vi "Test FFT time.vi"() -> ()   [LabVIEW 2018]
uses:
  General/type defines/FFT parameters.ctl
  <vilib>/Analysis/4window.llb/windowTd.ctl
  <vilib>/Analysis/NI_AALPro.lvlib
panel:
  out "Waveform Chart":sgl[][](graph)
  in  "error in (no error)":errorcluster
  out "time for FFT":dbl
  in  "FFT parameters":T1={"window"=1, "view"={"dB On (F)"=FALSE, "unwrap phase (F)"=FALSE, "convert to degree (F)"=FALSE}, "#A-lines"=2048, "start pixel"=0, "#pixels to save"=300} {"window" items=["Rectangle"=0, "Hanning"=1, "Hamming"=2, "Blackman-Harris"=3, "Exact Blackman"=4, "Blackman"=5, "Flat Top"=6, "4 Term B-Harris "=7, "7 Term B-Harris"=8, "Low Sidelobe"=9, "Blackman Nuttall"=11, "Triangle"=30, "Bartlett-Hanning"=31, "Bohman"=32, "Parzen"=33, "Welch"=34, "Kaiser"=60, "Dolph-Chebyshev"=61, "Gaussian"=62]}
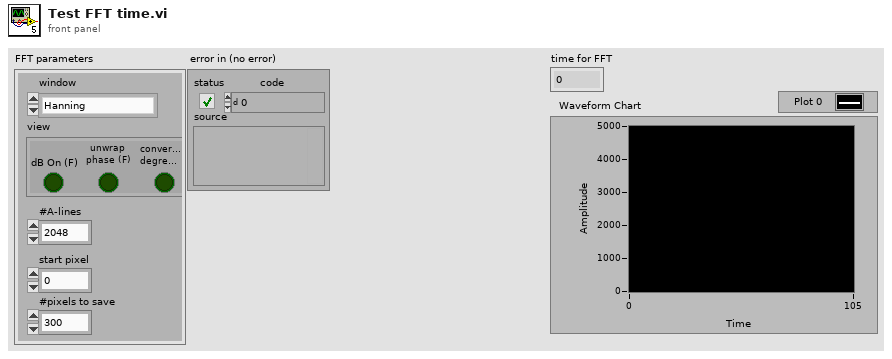
[diagram p1: front panel]
types:
  T1 = typedef "FFT parameters.ctl" = cluster{"window":T2, "view":cluster{"dB On (F)":bool, "unwrap phase (F)":bool, "convert to degree (F)":bool}, "#A-lines":i32, "start pixel":i32, "#pixels to save":i32}
  T2 = typedef "NI_AALPro.lvlib/windowTd.ctl" = u32
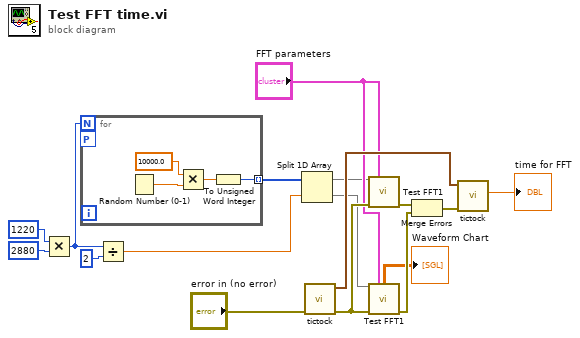
[diagram p0: block diagram]
diagram:
  n1 = Multiply(x=1220, y=2880) -> (x*y=w7:i32)
  n2 = for {
    N: w7 -> [_]
    tunnel: [w21] -> w4 mode=indexing
    workers-P: _ -> [_]
    n3 = Random Number (0-1)() -> (number: 0 to 1=w20:dbl)
    n4 = Multiply(x=10000.0, y=w20) -> (x*y=w18:dbl)
    n5 = To Unsigned Word Integer(number=w18) -> (unsigned 16bit integer=w21:u16)
  }
  n6 = Divide(x=w7, y=2) -> (x/y=w3:dbl)
  n7 = Split 1D Array(array=w4, index=w3) -> (first subarray=w2:u16[], second subarray=w1:u16[])
  n8 = call "tictock.vi"("error in (no error)"="error in (no error)") -> ("error out"=w12:errorcluster, "seconds since 1Jan1904"=w15:timestamp)  [unwired: 8 in, 1 out]
  n9 = call "Test FFT1.vi"("Buffer in"=w2, "FFT parameters"="FFT parameters", "error in"=w12) -> ("error out"=w10:errorcluster)  [unwired: 8 in, 4 out]
  n10 = call "Test FFT1.vi"("Buffer in"=w1, "FFT parameters"="FFT parameters", "error in"=w12) -> ("Mag for display"=→"Waveform Chart":sgl[][], "error out"=w11:errorcluster)  [unwired: 8 in, 3 out]
  n11 = Merge Errors(w10, w11) -> (w9:errorcluster)
  n12 = call "tictock.vi"("error in (no error)"=w9, "seconds since 1Jan1904 2"=w15) -> ("Numeric"=→"time for FFT":dbl)  [unwired: 7 in, 2 out]
